vi "Go To Executing.vi"(8 "error in (no error)":errorcluster, 11 "CommandStates In":refnum<class "Command State.lvclass">) -> (0 "error out":errorcluster, 3 "State out":refnum<class "State Actor.lvclass">)   [LabVIEW 2013, in "Command State.lvclass"]
uses:
  Command State.lvclass
  <vilib>/ni/Actors/State Actor/State Actor/State Actor.lvclass
  Executing/Executing.lvclass
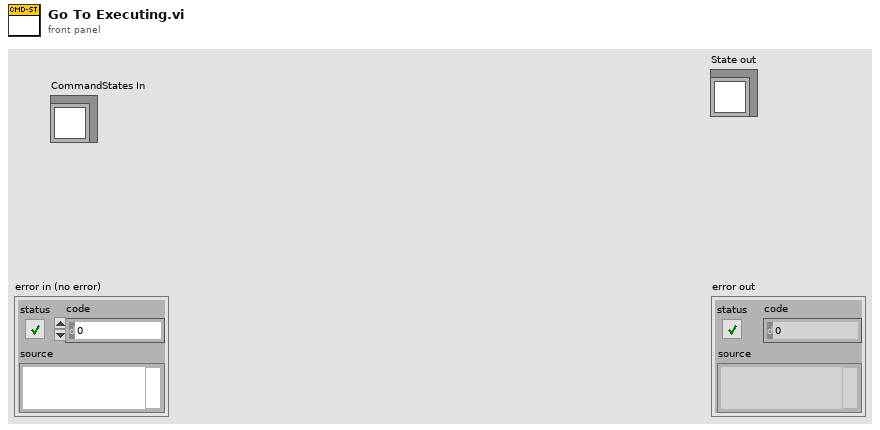
[diagram p1: front panel]
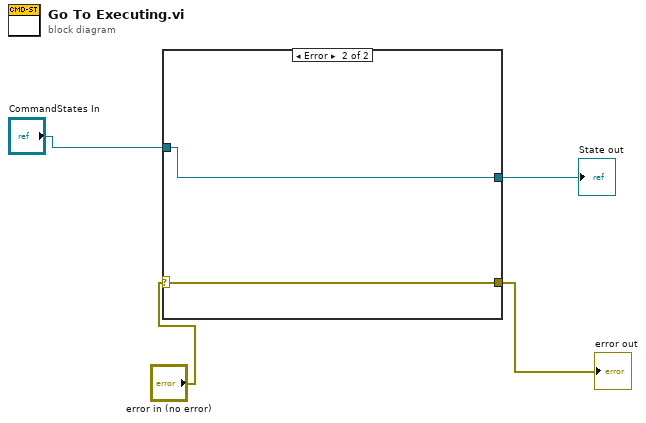
[diagram p0: block diagram]
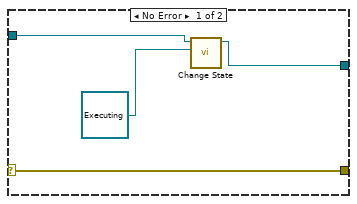
[diagram p2: hidden frame]
diagram:
  n1 = case shown="Error" "error in (no error)" {
    selector: "error in (no error)" -> [w8 w9]
    tunnel: [w8 w9] -> w3
    tunnel: "CommandStates In" -> [w7 w10]
    tunnel: [w5 w10] -> w1
    frame No Error {
      n2 = call <vilib>:"Change State.vi"("New State in"=refnum<class "Executing.lvclass"> refnum ("Command.lvlib:Executing.lvclass"), "State in"=w7) -> ("State out"=w5:refnum<class "State Actor.lvclass">)  [unwired: 8 in, 1 out]
    }
    frame Error {
    }
  }
  "error out" <- w3
  "State out" <- w1
